vi "Colour.vi"() -> ()   [LabVIEW 2022 SP3]
uses:
  <vilib>/DAQmx/read.llb/DAQmx Read (Analog DBL 1Chan 1Samp).vi
  <vilib>/DAQmx/write.llb/DAQmx Write (Digital Bool 1Line 1Point).vi
  <vilib>/DAQmx/create/channels.llb/DAQmx Create Channel (DO-Digital Output).vi
  <vilib>/DAQmx/miscellaneous.llb/DAQmx Fill In Error Info.vi
  <vilib>/DAQmx/create/channels.llb/DAQmx Create Channel (AI-Voltage-Basic).vi
  Reading Red.vi
  Reading Green.vi
  Reading Blue.vi
panel:
  out "[2]":dbl
  out "[1]":dbl
  out "[0]":dbl
  out "error out 4":errorcluster
  out "error out 3":errorcluster
  out "error out 2":errorcluster
  out "error out":errorcluster
  out "Array":dbl[](array[numeric])
  out "Numeric 2":i32
  out "red":bool
  out "blue":bool
  out "green":bool
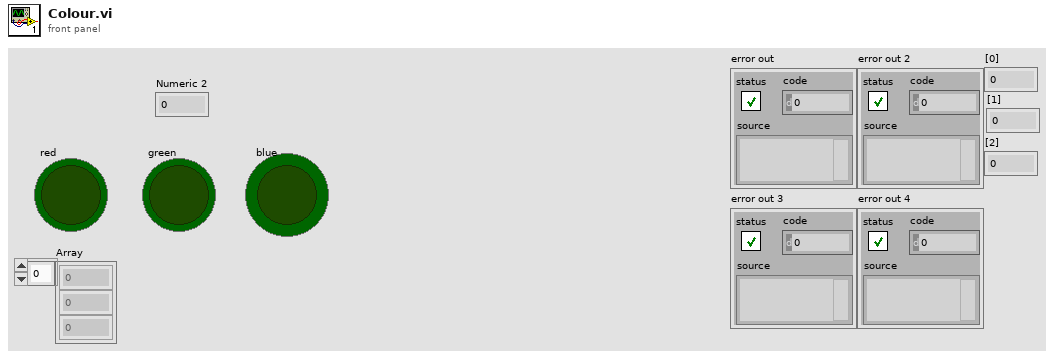
[diagram p1: front panel]
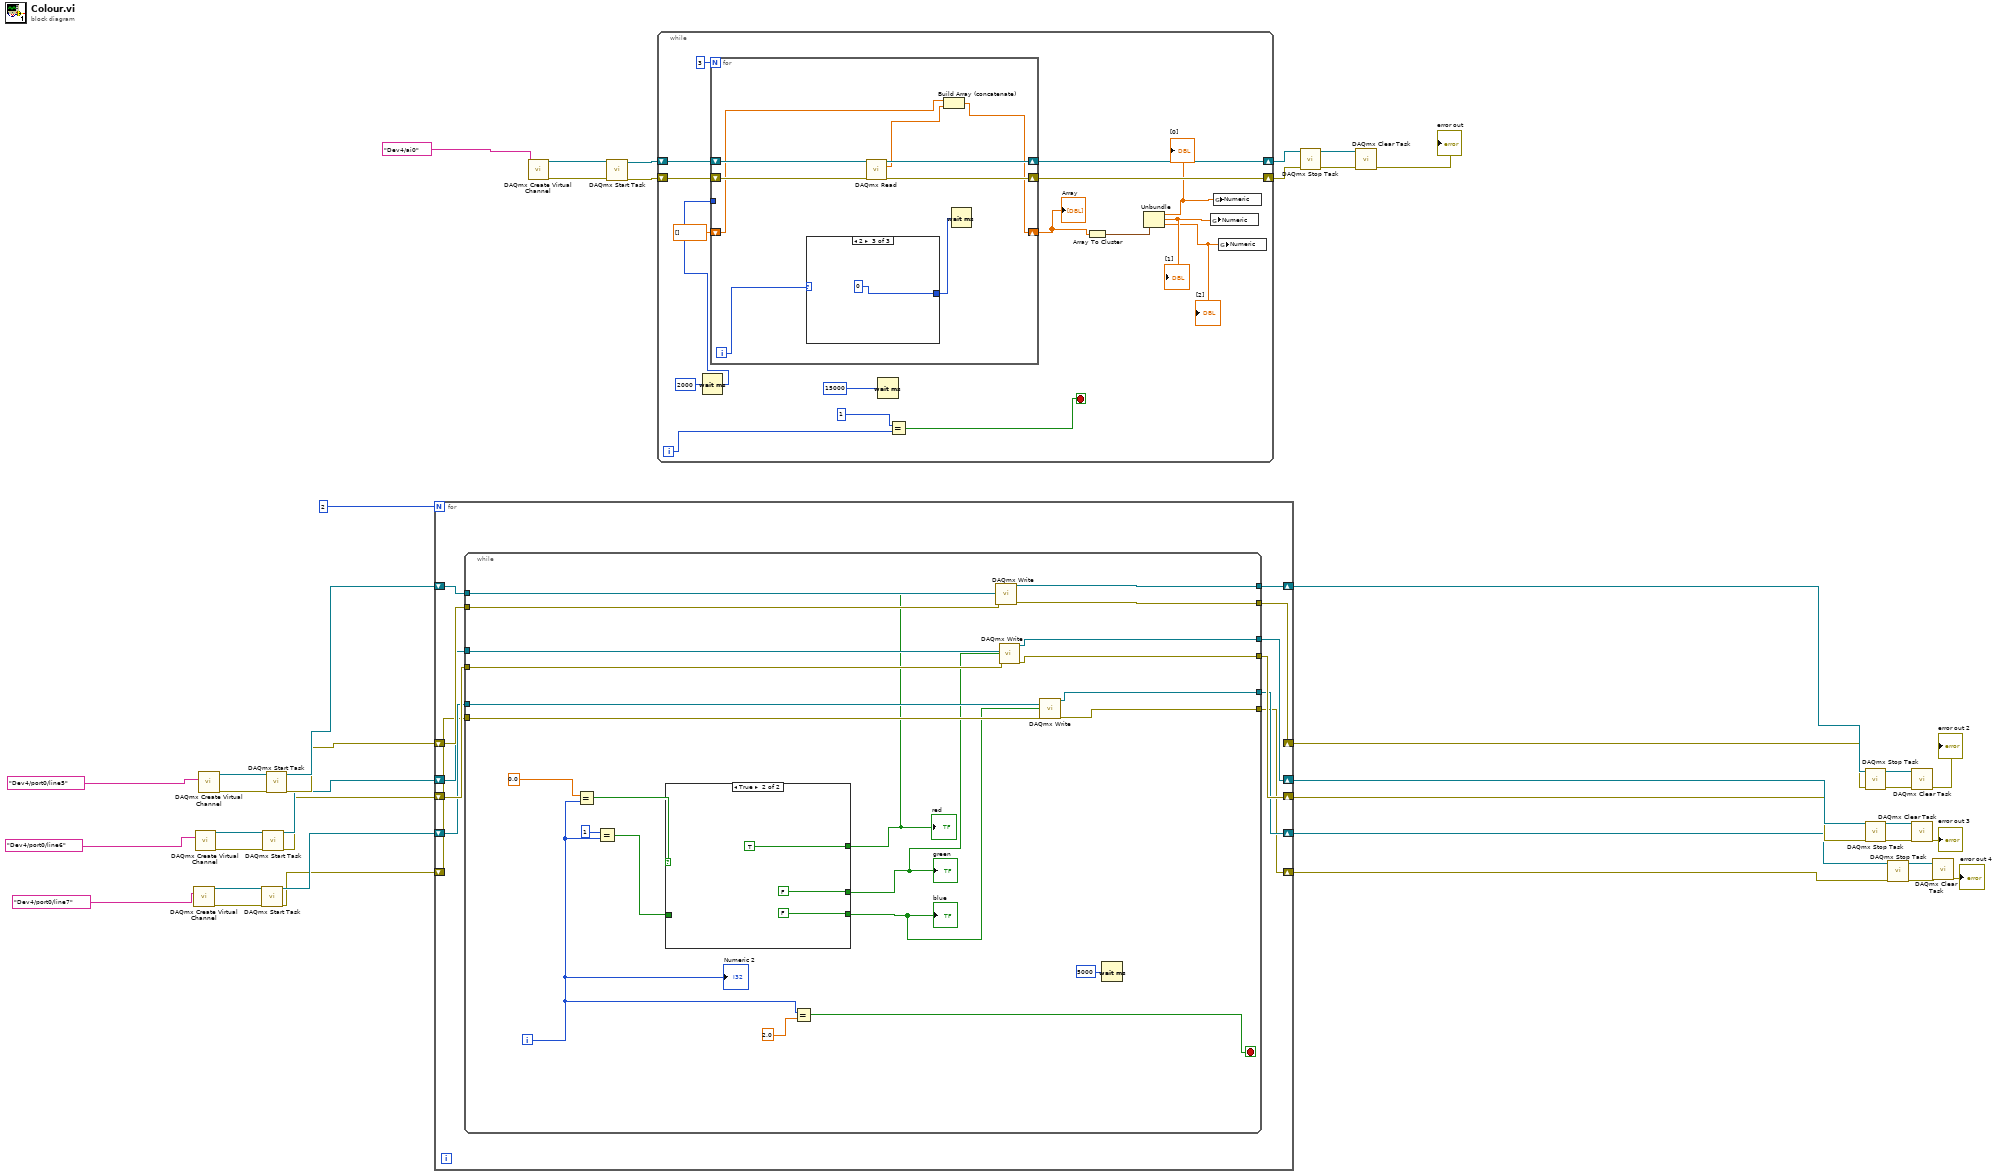
[diagram p0: block diagram]
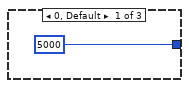
[diagram p2: hidden frame]
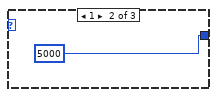
[diagram p3: hidden frame]
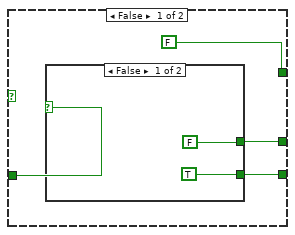
[diagram p4: hidden frame]
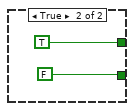
[diagram p5: hidden frame]
diagram:
  n1 = call-poly <vilib>:"DAQmx Create Virtual Channel.vi"("lines"=tag "Dev4/port0/line7" ("Blue Channel")) -> ("task out"=w32:refnum<k21>, "error out"=w33:errorcluster)  [unwired: 13 in]
  n2 = call-poly <vilib>:"DAQmx Create Virtual Channel.vi"("lines"=tag "Dev4/port0/line6" ("Green Channel")) -> ("task out"=w36:refnum<k21>, "error out"=w37:errorcluster)  [unwired: 13 in]
  n3 = call-poly <vilib>:"DAQmx Create Virtual Channel.vi"("lines"=tag "Dev4/port0/line5" ("Red Channel")) -> ("task out"=w40:refnum<k21>, "error out"=w41:errorcluster)  [unwired: 13 in]
  n4 = call <vilib>:"DAQmx Start Task.vi"("task/channels in"=w32, "error in"=w33) -> ("task out"=w22:refnum<k21>, "error out"=w21:errorcluster)  [unwired: 12 in]
  n5 = call <vilib>:"DAQmx Start Task.vi"("task/channels in"=w36, "error in"=w37) -> ("task out"=w24:refnum<k21>, "error out"=w23:errorcluster)  [unwired: 12 in]
  n6 = call <vilib>:"DAQmx Start Task.vi"("task/channels in"=w40, "error in"=w41) -> ("task out"=w26:refnum<k21>, "error out"=w25:errorcluster)  [unwired: 12 in]
  n7 = for {
    N: 2 -> [_]
    shift-right: [w47] -> w20
    shift-left: w26 -> [w53]
    shift-right: [w46] -> w19
    shift-left: w25 -> [w52]
    shift-right: [w45] -> w18
    shift-left: w24 -> [w51]
    shift-right: [w44] -> w17
    shift-left: w23 -> [w50]
    shift-right: [w43] -> w16
    shift-left: w22 -> [w49]
    shift-right: [w42] -> w15
    shift-left: w21 -> [w48]
    n8 = while {
      tunnel: w53 -> [w68]
      tunnel: w52 -> [w67]
      tunnel: [w66] -> w47
      tunnel: [w65] -> w46
      tunnel: w51 -> [w64]
      tunnel: w50 -> [w63]
      tunnel: [w62] -> w45
      tunnel: [w61] -> w44
      tunnel: w49 -> [w60]
      tunnel: w48 -> [w59]
      tunnel: [w58] -> w43
      tunnel: [w57] -> w42
      i -> [w70]
      stop <- w75 stop-if-true
      n9 = Equal?(x=0.0, y=w70) -> (x = y?=w72:bool)
      n10 = Equal?(x=1, y=w70) -> (x = y?=w71:bool)
      n11 = case shown="True" w72 {
        tunnel: [FALSE TRUE] -> w56
        tunnel: w71 -> [w80 _]
        tunnel: [w78 FALSE] -> w54
        tunnel: [w77 FALSE] -> w55
        frame False {
          n12 = case shown="False" w80 {
            tunnel: [FALSE TRUE] -> w78
            tunnel: [TRUE FALSE] -> w77
            frame False {
            }
            frame True {
            }
          }
        }
        frame True {
        }
      }
      "red" <- w56
      "blue" <- w55
      "green" <- w54
      n13 = Equal?(x=w70, y=2.0) -> (x = y?=w75:bool)
      n14 = call-poly <vilib>:"DAQmx Write.vi"("task/channels in"=w68, "data"=w56, "error in"=w67) -> ("task out"=w66:refnum<k21>, "error out"=w65:errorcluster)  [unwired: 10 in, 1 out]
      n15 = call-poly <vilib>:"DAQmx Write.vi"("task/channels in"=w64, "data"=w54, "error in"=w63) -> ("task out"=w62:refnum<k21>, "error out"=w61:errorcluster)  [unwired: 10 in, 1 out]
      n16 = call-poly <vilib>:"DAQmx Write.vi"("task/channels in"=w60, "data"=w55, "error in"=w59) -> ("task out"=w58:refnum<k21>, "error out"=w57:errorcluster)  [unwired: 10 in, 1 out]
      n17 = Wait (ms)(milliseconds to wait=u32 5000) -> ()  [unwired: 1 out]
      "Numeric 2" <- w70
    }
  }
  n18 = call-poly <vilib>:"DAQmx Create Virtual Channel.vi"("physical channels"=tag "Dev4/ai0") -> ("task out"=w12:refnum<k21>, "error out"=w13:errorcluster)  [unwired: 13 in]
  n19 = call <vilib>:"DAQmx Start Task.vi"("task/channels in"=w12, "error in"=w13) -> ("task out"=w9:refnum<k21>, "error out"=w8:errorcluster)  [unwired: 12 in]
  n20 = while {
    shift-right: [w102] -> w7
    shift-left: w9 -> [w104]
    shift-right: [w101] -> w6
    shift-left: w8 -> [w103]
    i -> [w93]
    stop <- w91 stop-if-true
    n21 = Wait (ms)(milliseconds to wait=u32 2000) -> (millisecond timer value=w97:u32)
    n22 = for {
      N: 3 -> [_]
      shift-right: [w111] -> w102
      shift-left: w104 -> [w113]
      shift-right: [w110] -> w101
      shift-left: w103 -> [w112]
      shift-right: [w106] -> w95
      shift-left: dbl[] [] -> [w108]
      tunnel: w97 -> [_]
      i -> [w109]
      n23 = case shown="2" w109 {
        tunnel: [u32 5000 ("milliseconds to wait") u32 5000 ("milliseconds to wait") u32 0 ("milliseconds to wait")] -> w105
        frame 0, Default {
        }
        frame 1 {
        }
        frame 2 {
        }
      }
      n24 = call-poly <vilib>:"DAQmx Read.vi"("task/channels in"=w113, "error in"=w112) -> ("task out"=w111:refnum<k21>, "data"=w107:dbl, "error out"=w110:errorcluster)  [unwired: 11 in]
      n25 = Build Array (concatenate)(w108, w107) -> (w106:dbl[])
      n26 = Wait (ms)(milliseconds to wait=w105) -> ()  [unwired: 1 out]
    }
    "Array" <- w95
    n27 = Wait (ms)(milliseconds to wait=u32 15000 ("millisecond timer value")) -> ()  [unwired: 1 out]
    n28 = Equal?(x=1, y=w93) -> (x = y?=w91:bool)
    n29 = Array To Cluster(array=w95) -> (cluster=w94:cluster{"[0]":dbl, "[1]":dbl, "[2]":dbl})
    n30 = Unbundle "Unbundle"(w94) -> ("[0]"=w89:dbl, "[1]"=w90:dbl, "[2]"=w88:dbl)
    "[0]" <- w89
    "[1]" <- w90
    "[2]" <- w88
    n31 = global write "Reading Green.vi" "Numeric"(w90) -> ()
    n32 = global write "Reading Red.vi" "Numeric"(w89) -> ()
    n33 = global write "Reading Blue.vi" "Numeric"(w88) -> ()
  }
  n34 = call <vilib>:"DAQmx Stop Task.vi"("task/channels in"=w7, "error in"=w6) -> ("task out"=w11:refnum<k21>, "error out"=w10:errorcluster)  [unwired: 12 in]
  n35 = call <vilib>:"DAQmx Clear Task.vi"("task in"=w11, "error in"=w10) -> ("error out"=→"error out":errorcluster)  [unwired: 13 in]
  n36 = call <vilib>:"DAQmx Stop Task.vi"("task/channels in"=w20, "error in"=w19) -> ("task out"=w39:refnum<k21>, "error out"=w38:errorcluster)  [unwired: 12 in]
  n37 = call <vilib>:"DAQmx Stop Task.vi"("task/channels in"=w18, "error in"=w17) -> ("task out"=w35:refnum<k21>, "error out"=w34:errorcluster)  [unwired: 12 in]
  n38 = call <vilib>:"DAQmx Stop Task.vi"("task/channels in"=w16, "error in"=w15) -> ("task out"=w31:refnum<k21>, "error out"=w30:errorcluster)  [unwired: 12 in]
  n39 = call <vilib>:"DAQmx Clear Task.vi"("task in"=w39, "error in"=w38) -> ("error out"=→"error out 2":errorcluster)  [unwired: 13 in]
  n40 = call <vilib>:"DAQmx Clear Task.vi"("task in"=w35, "error in"=w34) -> ("error out"=→"error out 3":errorcluster)  [unwired: 13 in]
  n41 = call <vilib>:"DAQmx Clear Task.vi"("task in"=w31, "error in"=w30) -> ("error out"=→"error out 4":errorcluster)  [unwired: 13 in]
